vi "VelocityControl.vi"(0 "estimatives":T3, 1 "Dest_orientation":dbl, 2 "Position":dbl[](array[numeric]), 3 "Waypoint 1":dbl[](array[numeric]), 4 "Waypoint 0":dbl[](array[numeric]), 5 "Vx":dbl format="%#_13g", 9 "Vy":dbl format="%#_13g", 10 "PID Gains Angle":T2={"proportional gain (Kc)"=5.0, "integral time (Ti, min)"=0.0, "derivative time (Td, min)"=-2.0}, 11 "output xy":dbl=2.4, 12 "output inc":dbl=2.4, 13 "output angle":dbl=4.0, 14 "PID gains Vel":T2={"proportional gain (Kc)"=0.6, "integral time (Ti, min)"=0.0, "derivative time (Td, min)"=0.0}, 15 "PID Gains lateral":T2={"proportional gain (Kc)"=0.1, "integral time (Ti, min)"=0.0, "derivative time (Td, min)"=0.0}) -> (8 "Output Velocity":dbl[](array[numeric]) format="%.2f")   [LabVIEW 2018]
uses:
  Controle/VelocityGraph.ctl
  <vilib>/Analysis/coordinate.llb/Wrap Angle (scalar).vi
  <vilib>/Analysis/coordinate.llb/2D Cartesian Coordinate Rotation (Scalar).vi
  <vilib>/Analysis/NI_AAL_Angle.lvlib
  <vilib>/Analysis/NI_AALPro.lvlib
panel:
  out "Velocity Y":T1
  out "Velocity X":T1
  in  "Reinitialize":bool
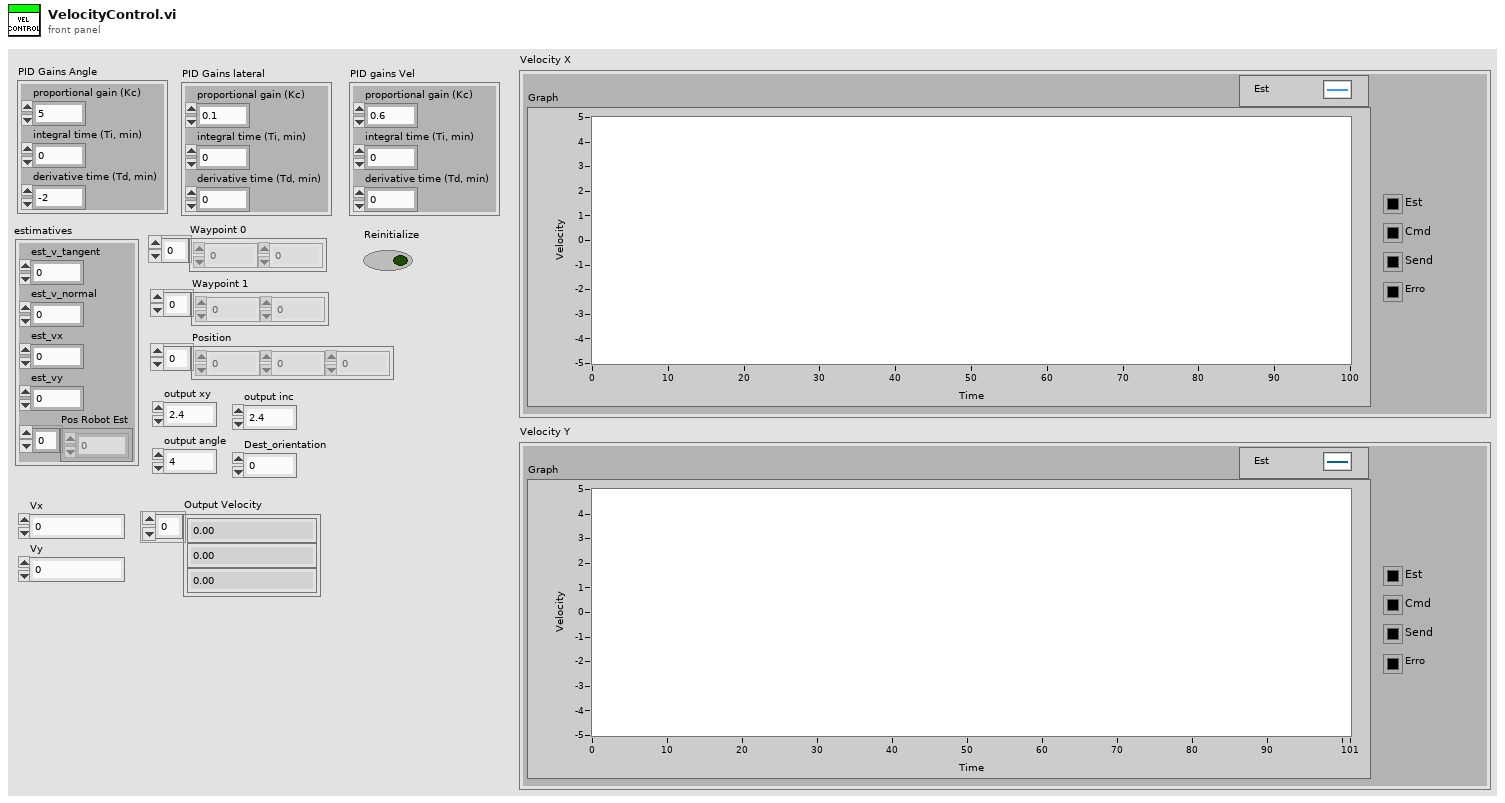
[diagram p1: front panel]
types:
  T1 = typedef "VelocityGraph.ctl" = cluster{"Graph":cluster{"est_vx":dbl, "Vx":dbl, dbl, "x out":dbl}, "Est":u32, "Cmd":u32, "Send":u32, "Erro":u32}
  T2 = cluster{"proportional gain (Kc)":dbl, "integral time (Ti, min)":dbl, "derivative time (Td, min)":dbl}
  T3 = cluster{"est_v_tangent":dbl, "est_v_normal":dbl, "est_vx":dbl, "est_vy":dbl, "Pos Robot Est":dbl[]}
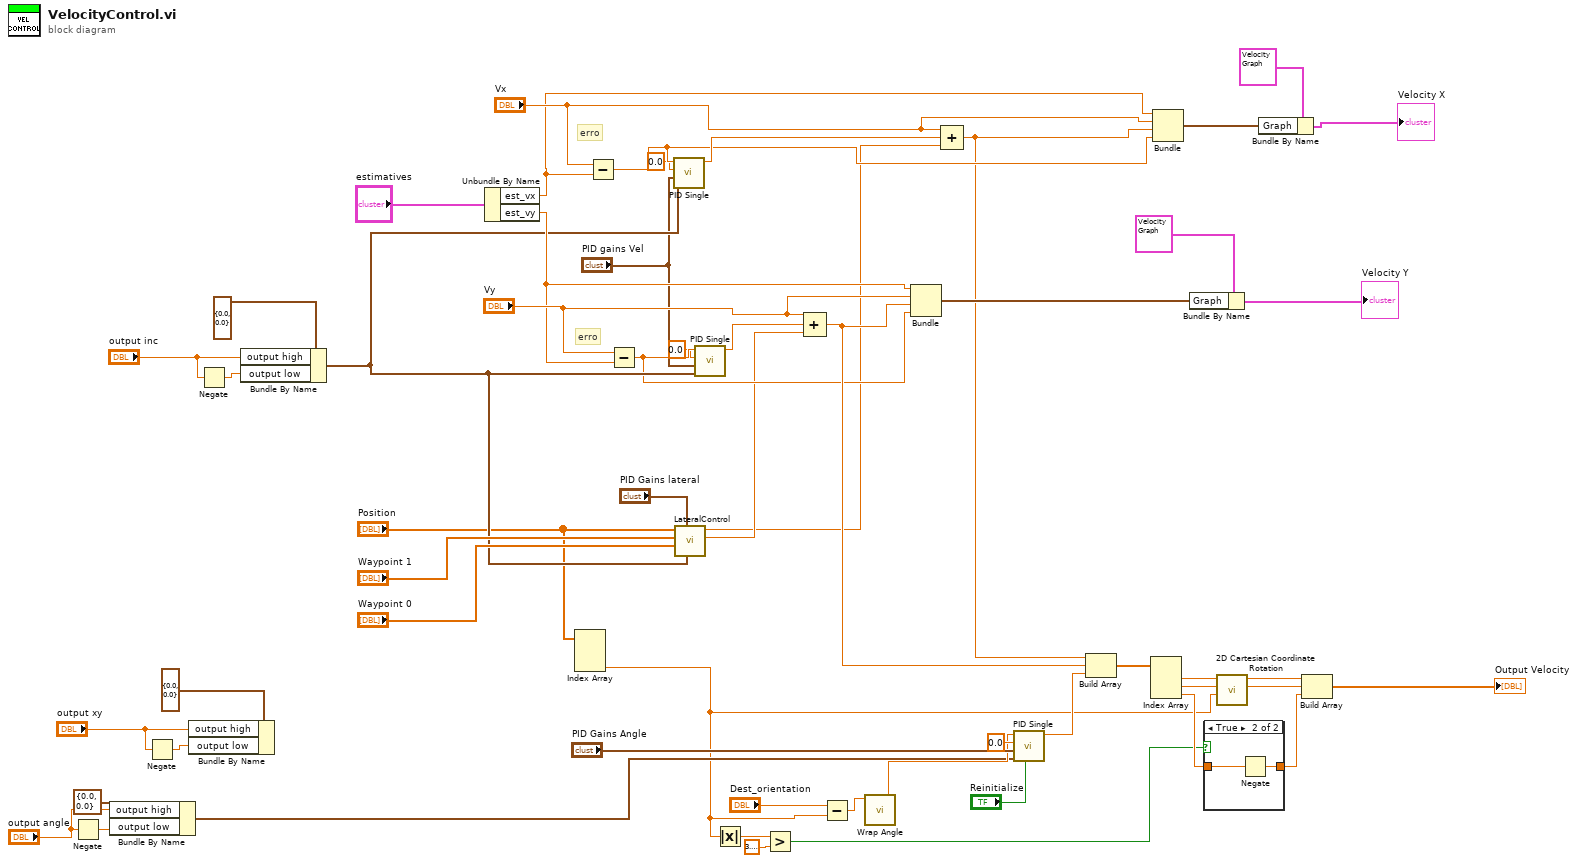
[diagram p0: block diagram]
diagram:
  # "erro"
  # "erro"
  n1 = Negate(x="output angle") -> (-x=w37:dbl)
  n2 = Bundle By Name(cluster=cluster{"output high":dbl, "output low":dbl} {"output high"=0.0, "output low"=0.0}, "output high"="output angle", "output low"=w37) -> (w12:cluster{"output high":dbl, "output low":dbl})
  n3 = Negate(x="output xy") -> (-x=w39:dbl)
  n4 = Bundle By Name(cluster=cluster{"output high":dbl, "output low":dbl} {"output high"=0.0, "output low"=0.0} ("new element/subarray"), "output high"="output xy", "output low"=w39) -> ()  [unwired: 1 out]
  n5 = Negate(x="output inc") -> (-x=w22:dbl)
  n6 = Bundle By Name(cluster=cluster{"output high":dbl, "output low":dbl} {"output high"=0.0, "output low"=0.0} ("new element/subarray"), "output high"="output inc", "output low"=w22) -> (w11:cluster{"output high":dbl, "output low":dbl})
  n7 = Unbundle By Name("estimatives") -> ("est_vx"=w20:dbl, "est_vy"=w19:dbl)
  n8 = Index Array(array="Position") -> (element #3=w9:dbl)  [unwired: 3 in, 2 out]
  n9 = Subtract(x="Vx", y=w20) -> (x-y=w8:dbl)
  n10 = Subtract(x="Vy", y=w19) -> (x-y=w6:dbl)
  n11 = call "PID Single.vi"("Limits"=w11, "PID gains in"="PID gains Vel", "Variable"=0.0 ("Setpoint"), "Setpoint"=w8) -> ("Out"=w28:dbl)  [unwired: 7 in]
  n12 = call "LateralControl.vi"("output range"=w11, "PID Gains lateral"="PID Gains lateral", "Waypoint 0"="Waypoint 0", "Waypoint 1"="Waypoint 1", "Position"="Position") -> ("y out"=w3:dbl, "x out"=w2:dbl)  [unwired: 5 in]
  n13 = call "PID Single.vi"("Limits"=w11, "PID gains in"="PID gains Vel", "Variable"=0.0 ("Setpoint"), "Setpoint"=w6) -> ("Out"=w27:dbl)  [unwired: 7 in]
  n14 = Absolute Value(x=w9) -> (abs(x)=w52:dbl)
  n15 = Greater?(x=w52, y=3.141592653589793) -> (0:w47:bool)
  n16 = Compound Arithmetic op=ADD("Vy", w27, w3) -> (w24:dbl)
  n17 = Subtract(x="Dest_orientation", y=w9) -> (x-y=w44:dbl)
  n18 = call-poly <vilib>:"Wrap Angle.vi"("angle in"=w44) -> ("angle out"=w43:dbl)  [unwired: 9 in, 1 out]
  n19 = Bundle("est_vy"=w19, "Vy"="Vy", w24, w6) -> (w17:cluster{"est_vy":dbl, "Vy":dbl, dbl, dbl})  [unwired: 1 in]
  n20 = Compound Arithmetic op=ADD("Vx", w28, w2) -> (w1:dbl)
  n21 = call "PID Single.vi"("initialize"="Reinitialize", "Limits"=w12, "PID gains in"="PID Gains Angle", "Variable"=0.0, "Setpoint"=w43) -> ("Out"=w48:dbl)  [unwired: 6 in]
  n22 = Build Array(w1, w24, w48) -> (w42:dbl[])
  n23 = Index Array(array=w42) -> (element #1=w56:dbl, element #2=w55:dbl, element #3=w51:dbl)  [unwired: 3 in]
  n24 = Bundle("est_vx"=w20, "Vx"="Vx", w1, w8) -> (w14:cluster{"est_vx":dbl, "Vx":dbl, dbl, dbl})  [unwired: 1 in]
  n25 = Bundle By Name(cluster=T1 {"Graph"={"est_vx"=-0.14571416207204627, "Vx"=0.4692407651588243, 1.5797768746041183, "x out"=1.110536109445294}, "Est"=16860, "Cmd"=16711680, "Send"=6618880, "Erro"=16776722} ("Velocity Y"), "Graph"=w17) -> (→"Velocity Y":T1)
  n26 = case shown="True" w47 {
    tunnel: w51 -> [w57 w59]
    tunnel: [w57 w58] -> w50
    frame False {
    }
    frame True {
      n27 = Negate(x=w59) -> (-x=w58:dbl)
    }
  }
  n28 = call-poly <vilib>:"2D Cartesian Coordinate Rotation.vi"("theta"=w9, "y"=w55, "x"=w56) -> ("y out"=w53:dbl, "x out"=w54:dbl)  [unwired: 6 in, 1 out]
  n29 = Bundle By Name(cluster=T1 {"Graph"={"est_vx"=-0.14571416207204627, "Vx"=0.4692407651588243, 1.5797768746041183, "x out"=1.110536109445294}, "Est"=16860, "Cmd"=16711680, "Send"=6618880, "Erro"=16776722} ("Velocity Y"), "Graph"=w14) -> (→"Velocity X":T1)
  n30 = Build Array(w54, w53, w50) -> (→"Output Velocity":dbl[])
